vi "loop.vi"() -> ()   [LabVIEW 2017]
uses:
  <vilib>/FPGAPlugInAG/myRIO-1900/niLvFpga_Open_myRIO-1900.vi
  <vilib>/rvi/interface/common/dynamic/niFpgaDynamicAddResources.vi
  <vilib>/Utility/error.llb/Error Cluster From Error Code.vi
  <vilib>/rvi/errors/niLvFpgaAdjustHostInterfaceError.vi
  <vilib>/FPGAPlugInAG/Dynamic/niLvFpga_Close_Dynamic.vi
  <vilib>/rvi/interface/nirviOpenFPGA/nirviOpenFPGA.xnode
  FPGA Bitfiles/test-3-dcdccontr_FPGATarget_FPGAcontroller_wkO7c1aMSH4.lvbitx
  FPGA_controller.vi
  <vilib>/rvi/interface/nirviReadWriteControl/nirviReadWriteControl.xnode
  <vilib>/rvi/interface/nirviCloseFPGA/nirviCloseFPGA.xnode
  NiFpgaLv.dll
  <vilib>/rvi/interface/Simulation/niFpgaSimulationCallBeginRW.vi
panel:
  out "Iteration":i32
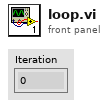
[diagram p1: front panel]
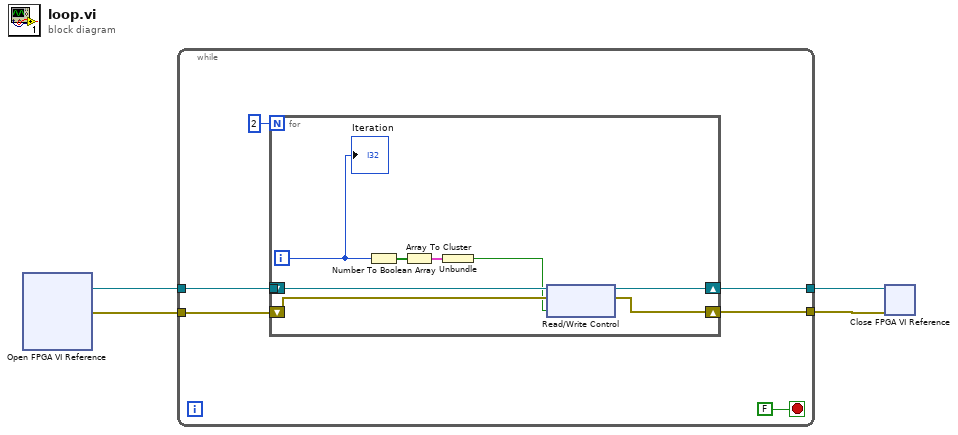
[diagram p0: block diagram]
diagram:
  n1 = xnode "Open FPGA VI Reference"() -> ("FPGA VI Reference Out"=w4:refnum<k20>, "error out"=w3:errorcluster)  [unwired: 2 in]
  n2 = while {
    tunnel: w4 -> [w8]
    tunnel: w3 -> [w7]
    tunnel: [w6] -> w2
    tunnel: [w5] -> w1
    stop <- FALSE stop-if-true
    n3 = for {
      N: 2 -> [_]
      tunnel: w8 -> [w15]
      shift-right: [w13] -> w6
      shift-left: _ -> [_]
      shift-right: [w12] -> w5
      shift-left: w7 -> [w14]
      i -> [w16]
      n4 = Number To Boolean Array(number=w16) -> (Boolean array=w18:bool[])
      n5 = Array To Cluster(array=w18) -> (cluster=w17:cluster{"Boolean array[0]":bool})
      n6 = Unbundle(w17) -> ("Boolean array[0]"=w11:bool)
      n7 = xnode "Read/Write Control"("FPGA VI Reference In"=w15, "error in"=w14, "Input test"=w11) -> ("FPGA VI Reference Out"=w13:refnum<k20>, "error out"=w12:errorcluster)
      "Iteration" <- w16
    }
  }
  n8 = xnode "Close FPGA VI Reference"("FPGA VI Reference In"=w2, "error in"=w1) -> ()  [unwired: 1 out]
